vi "string-unbundler-1.vi"(1 "String":string) -> (0 "Array 1":dbl[](array[numeric]))   [LabVIEW 2023]
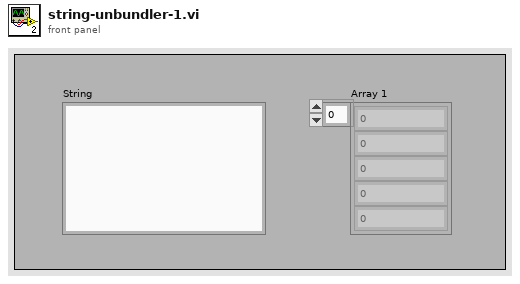
[diagram p1: front panel]
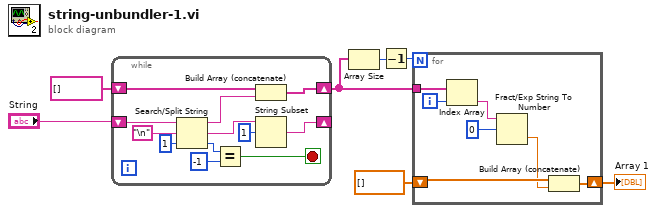
[diagram p0: block diagram]
diagram:
  n1 = while {
    shift-right: [w16] -> w7
    shift-left: string[] [] -> [w18]
    shift-right: [w10] -> _
    shift-left: "String" -> [w17]
    stop <- w13 stop-if-true
    n2 = Search/Split String(string=w17, search string/char (-)="\n", offset (0)=1) -> (substring before match=w19:string, match + rest of string=w11:string, offset of match=w15:i32)
    n3 = Equal?(x=w15, y=-1) -> (x = y?=w13:bool)
    n4 = Build Array (concatenate)(w18, w19) -> (w16:string[])
    n5 = String Subset(string=w11, offset (0)=1) -> (substring=w10:string)  [unwired: 1 in]
  }
  n6 = Array Size(array=w7) -> (size(s)=w1:i32)
  n7 = Decrement(x=w1) -> (x-1=w2:i32)
  n8 = for {
    N: w2 -> [_]
    tunnel: w7 -> [w26]
    shift-right: [w23] -> w4
    shift-left: dbl[] [] -> [w24]
    i -> [w25]
    n9 = Index Array(array=w26, index=w25) -> (element=w21:string)
    n10 = Fract/Exp String To Number(string=w21, offset=0) -> (number=w20:dbl)  [unwired: 2 in, 1 out]
    n11 = Build Array (concatenate)(w24, w20) -> (w23:dbl[])
  }
  "Array 1" <- w4
